vi "Encoder Read.vi"(0 "Arduino Resource":T1={"VISA resource"="COM11", "Board Type"=enum."Uno", "Connection Type"=enum."USB / Serial", "Bytes Per Packet (15)"=15}, 7 "Encoder Number (0)":u8, 11 "error in":errorcluster) -> (4 "Arduino Resource Out":T1={"VISA resource"="COM11", "Board Type"=enum."Uno", "Connection Type"=enum."USB / Serial", "Bytes Per Packet (15)"=15}, 8 "Count":i32, 15 "error out":errorcluster)   [LabVIEW 2018]
doc: "Read encoder value from Arduino.\nArduino Mega 2560 pin pairs to use for encoders (0, 1, 2) are 2 & 3, 18 & 19, 20 & 21.\nArduino Uno only has one pair of pins, 2 & 3 (encoder index 0).\nMust use the custom encoder version of the LIFA firmware."
uses:
  <vilib>/LabVIEW Interface for Arduino/Type Defs/Arduino Resource.ctl
  <vilib>/LabVIEW Interface for Arduino/Type Defs/Board Type.ctl
  <vilib>/LabVIEW Interface for Arduino/LabVIEW Interface for Arduino.lvlib
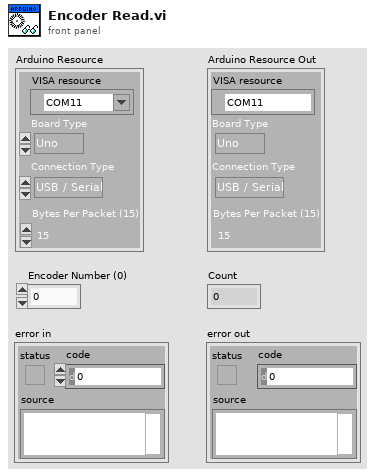
[diagram p1: front panel]
types:
  T1 = typedef "LabVIEW Interface for Arduino.lvlib/Arduino Resource.ctl" = cluster{"VISA resource":refnum<visa-resource-name>, "Board Type":T2, "Connection Type":enum8{"USB / Serial"}, "Bytes Per Packet (15)":u8}
  T2 = typedef "LabVIEW Interface for Arduino.lvlib/Board Type.ctl" = enum16{"Uno", "Dimuelanove w/Atmega 328", "Mega 2560"}
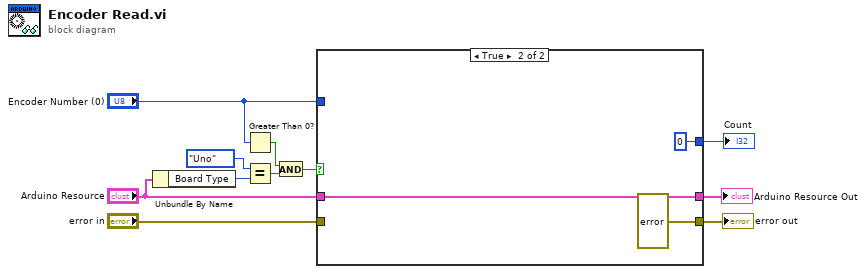
[diagram p0: block diagram]
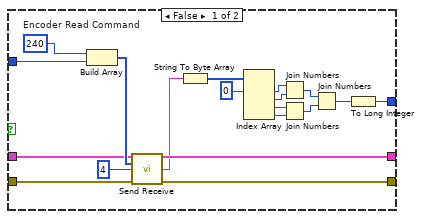
[diagram p2: hidden frame]
diagram:
  n1 = Unbundle By Name("Arduino Resource") -> ("Board Type"=w6:T2)
  n2 = Greater Than 0?(x="Encoder Number (0)") -> (x > 0?=w3:bool)
  n3 = Equal?(x=Board_Type."Uno", y=w6) -> (x = y?=w2:bool)
  n4 = And(x=w3, y=w2) -> (x .and. y?=w1:bool)
  n5 = case shown="True" w1 {
    tunnel: [w30 w33] -> w11
    tunnel: [w29 errorcluster {"status"=TRUE, "code"=0, "source"="Arduino Uno only has one encoder (index 0)."} ("error out")] -> w10
    tunnel: "error in" -> [w28 _]
    tunnel: [w15 0] -> w8
    tunnel: "Arduino Resource" -> [w14 w33]
    tunnel: "Encoder Number (0)" -> [w13 _]
    frame False {
      w12 = u8 240  # Encoder Read Command
      n6 = Build Array(w12, w13) -> (w26:u8[])
      n7 = call <vilib>:"Send Receive.vi"("Arduino Resource"=w14, "Data"=w26, "Bytes To Read (0)"=u8 4, "error in"=w28) -> ("Arduino Resource"=w30:T1, "Read Buffer"=w25:string, "error out"=w29:errorcluster)  [unwired: 9 in]
      n8 = String To Byte Array(string=w25) -> (unsigned byte array=w21:u8[])
      n9 = Index Array(array=w21, index #1=0 ("index")) -> (element #1=w23:u8, element #2=w24:u8, element #3=w20:u8, element #4=w19:u8)  [unwired: 3 in]
      n10 = Join Numbers(hi=w23, lo=w24) -> ((hi.lo)=w17:u16)
      n11 = Join Numbers(hi=w20, lo=w19) -> ((hi.lo)=w18:u16)
      n12 = Join Numbers(hi=w17, lo=w18) -> ((hi.lo)=w16:u32)
      n13 = To Long Integer(number=w16) -> (32bit integer=w15:i32)
    }
    frame True {
    }
  }
  "error out" <- w10
  "Arduino Resource Out" <- w11
  "Count" <- w8
